vi "p1_Control_temperatura.vi"() -> ()   [LabVIEW 2019]
uses:
  Control_temp.ctl
panel:
  out "Sensor de temperatura en °C":dbl(slide) scale=0.0..100.0
  in  "Rata de T":T1=1.0 scale=0.0..10.0
  in  "Selector":bool
  # "Incrementar"
  # "Decrementar"
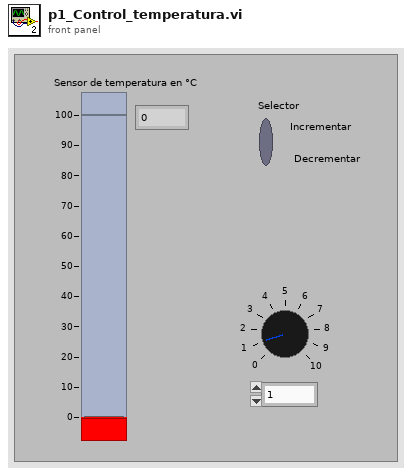
[diagram p1: front panel]
types:
  T1 = typedef "Control_temp.ctl" = dbl
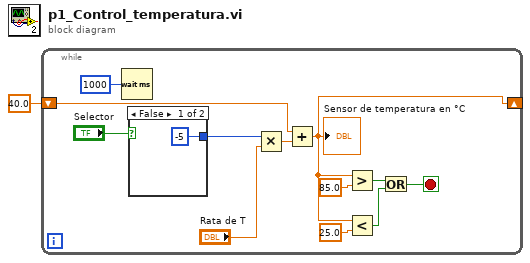
[diagram p0: block diagram]
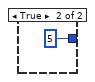
[diagram p2: hidden frame]
diagram:
  n1 = while {
    shift-right: [w3] -> _
    shift-left: T1 40.0 ("Rata de T") -> [w8]
    stop <- w5 stop-if-true
    n2 = Wait (ms)(milliseconds to wait=1000) -> ()  [unwired: 1 out]
    n3 = case shown="False" "Selector" {
      tunnel: [-5 5] -> w11
      frame False {
      }
      frame True {
      }
    }
    n4 = Multiply(x=w11, y="Rata de T") -> (x*y=w9:T1)
    n5 = Add(x=w8, y=w9) -> (x+y=w3:T1)
    "Sensor de temperatura en °C" <- w3
    n6 = Greater?(x=w3, y=85.0) -> (0:w7:bool)
    n7 = Less?(x=w3, y=T1 25.0) -> (x < y?=w6:bool)
    n8 = Or(x=w7, y=w6) -> (x .or. y?=w5:bool)
  }
